vi "Test FPGA.vi"() -> ()   [LabVIEW 2016]
uses:
  <vilib>/Platform/TimedLoop/XDataNode/timing_clust.ctl
  <vilib>/Platform/TimedLoop/XDataNode/nitl_modes.ctl
  <vilib>/Platform/TimedLoop/XDataNode/wakeup.ctl
  <vilib>/rvi/Emulation/niFpgaSctlEmulationGetInTimedLoop.vi
  <vilib>/rvi/Emulation/niFpgaEmulationReportErrorSimple.vi
  <vilib>/rvi/Emulation/niFpgaGetClockAttributes.vi
  <vilib>/rvi/Emulation/niFpgaCriticalErrorInLSC.vi
  <vilib>/rvi/Emulation/niFpgaProcessEmulError.vi
  <vilib>/RQC/FPGA Basic Logic/Counters/Counter (U8).vi
  <vilib>/rvi/Emulation/niFpgaEmulationIsFPGAContextNoSignature.vi
  <vilib>/rvi/DataTransferAndStorage/Container/Common/niFpgaContainerGetUniqueNameForEmu.vi
  <vilib>/rvi/Memory/Memory_Emulation/niFpgaMemoryEmulationCacheClearOnFirstRun.vi
  <vilib>/rvi/Memory/Memory_Emulation/nirvimemoryEmulationManagerCache_MakeExclusive.vi
  <vilib>/rvi/Memory/Memory_Emulation/niFpgaMemoryEmulationValidateCache.vi
  <vilib>/rvi/Memory/Memory_Emulation/nirvimemoryEmulationManagerCache_InsertValue.vi
  <vilib>/Utility/error.llb/Clear Errors.vi
  <vilib>/rvi/Memory/Memory_Emulation/nirvimemoryEmulationManagerCache_ReleaseExclusive.vi
  <vilib>/rvi/Memory/Memory_Emulation/nirvimemoryEmulationManagerCache_GetValue.vi
  <vilib>/rvi/Memory/Memory_Emulation/nirvimemoryEmulationManagerCache_SetValue.vi
  <vilib>/rvi/DataTransferAndStorage/Container/Common/niFpgaContainerSetEmuInfo.vi
  <vilib>/rvi/eio/common/nirviEmuReportErrorAndStop.vi
  <vilib>/RQC/FPGA Basic Logic/Counters/Counter (U32).vi
  <vilib>/Platform/TimedLoop/XDataNode/XDataNode.xnode
  <vilib>/rvi/DataTransferAndStorage/Container/XNode/niFpgaContainer.xnode
  <vilib>/rvi/DataTransferAndStorage/Register/Emulation/niFpgaRegisterEmulation.vi
  <vilib>/rvi/LocalResourceManager/LocalResourceManager.xnode
  <vilib>/Platform/TimedLoop/XDataNode/XDNodeRunTimeDep.lvlib
panel:
  in  "PD.max meas length":u32
  in  "detector signal in":bool
  in  "PD.reset":bool
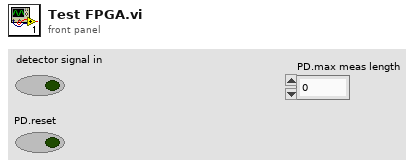
[diagram p1: front panel]
types:
  T1 = typedef "XDNodeRunTimeDep.lvlib/timing_clust.ctl" = cluster{"Expected End [f-1]":u64, "Actual End [f-1]":u64, "Finished Late? [f-1]":bool, "Expected End [i-1]":u64, "Actual End [i-1]":u64, "Finished Late? [i-1]":bool, "Expected Start [i]":u64, "Actual Start [i]":u64, "Expected Start [f]":u64, "Actual Start [f]":u64, "Source Name":string, "Structure Name":string, "Period":i64, "Deadline":i64, "Offset":i64, "Start":i64, "Priority":i32, "Timeout":i32, "Mode":T2, "Wakeup Reason":T3, "Error":errorcluster, "Source Type":string, "Secondary Source Type":string, "Global End Time":u64, "Global Start Time":u64, "Frame Duration":u64, "Iteration Duration":u64, "Assigned CPU":i32, "I/O Scan Engine Mode":u32}
  T2 = typedef "XDNodeRunTimeDep.lvlib/nitl_modes.ctl" = enum32{"No Change", "Process missed periods, maintain original phase", "Discard missed periods, maintain original phase", "Process missed periods, ignore original phase", "Discard missed periods, ignore original phase"}
  T3 = typedef "XDNodeRunTimeDep.lvlib/wakeup.ctl" = enum32{"Normal", "Aborted", "Asynchronous wakeup", "Timing source error", "Timed loop error", "Timeout"}
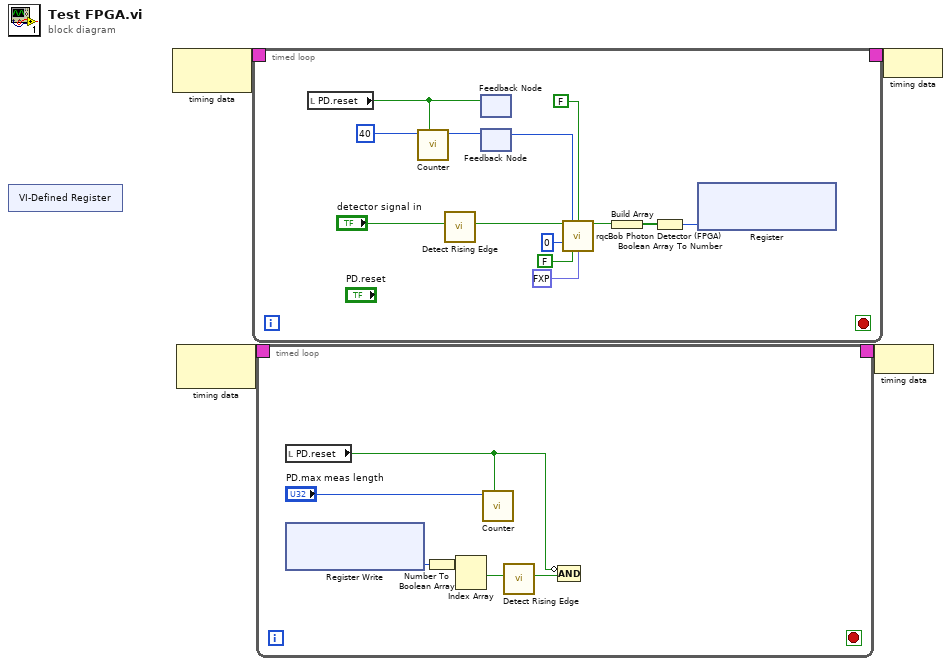
[diagram p0: block diagram]
diagram:
  n1 = xnode "VI-Defined Register"() -> ()  [unwired: 1 out]
  n2 = node-c288() -> (w4:T1)  [unwired: 1 in]
  n3 = node-c288() -> (w2:T1)  [unwired: 1 in]
  n4 = timed-loop {
    timing: w4 -> [_]
    timing-out: [_] -> w3
    stop <- _ stop-if-true
    n5 = local read "PD.reset"() -> (w17:bool)
    n6 = call-poly <vilib>:"Counter.vi"("reset"=w17, "bound"=u8 40 ("SPD.detection cycle length")) -> ("count out"=w16:u8)  [unwired: 8 in, 1 out]
    n7 = call <vilib>:"Detect Rising Edge.vi"("signal"="detector signal in") -> ("edge detected"=w6:bool)  [unwired: 10 in]
    n8 = feedback #1() -> ()  [unwired: 2 in]
    n9 = feedback-in #1(w17) -> ()
    n10 = feedback #2() -> (w14:u8)  [unwired: 1 in]
    n11 = feedback-in #2(w16) -> ()
    n12 = call "rqcBob Photon Detector (FPGA).vi"("detector signal in"=w6, "current cycle"=w14, "reset"=FALSE, "detector.detector window"=u16 0, "detector.use detector window"=FALSE, "detection pulse width"=fxp<+,4,4> 8.0) -> ("detector out"=w10:bool)  [unwired: 9 in]
    n13 = Build Array(w10) -> (w9:bool[])
    n14 = Boolean Array To Number(Boolean array=w9) -> (number=w8:u8)
    n15 = xnode "Register"("Data"=w8) -> ()  [unwired: 1 in, 1 out]
  }
  n16 = timed-loop {
    timing: w2 -> [_]
    timing-out: [_] -> w1
    stop <- _ stop-if-true
    n17 = local read "PD.reset"() -> (w22:bool)
    n18 = xnode ("Register Write")() -> ("Data"=w24:u8)  [unwired: 1 in, 1 out]
    n19 = Number To Boolean Array(number=w24) -> (Boolean array=w23:bool[])
    n20 = Index Array(array=w23) -> (element #1=w20:bool)  [unwired: 2 in, 1 out]
    n21 = call-poly <vilib>:"Counter.vi"("reset"=w22, "bound"="PD.max meas length") -> ()  [unwired: 8 in, 2 out]
    n22 = call <vilib>:"Detect Rising Edge.vi"("signal"=w20) -> ("edge detected"=w21:bool)  [unwired: 10 in]
    n23 = Compound Arithmetic op=AND(invert w22, w21) -> ()  [unwired: 1 out]
  }
  n24 = node-c288(w1) -> ()
  n25 = node-c288(w3) -> ()
